vi "cfg combine v2 and v32.vi"(8 "error in":errorcluster, 10 "Log Actions":T1(array[cluster]), 11 "Engine Configuration In":T3(array[cluster])) -> (0 "error out":errorcluster, 3 "Engine Configuration Out":T4[](array[typedef]))   [LabVIEW 2013, in "Standard Engine Configuration.lvclass"]
uses:
  Standard Engine Configuration.lvclass
  Module Specific Configuration.ctl
  Module Decimation.ctl
  Runtime/error responses.ctl
  error options.ctl
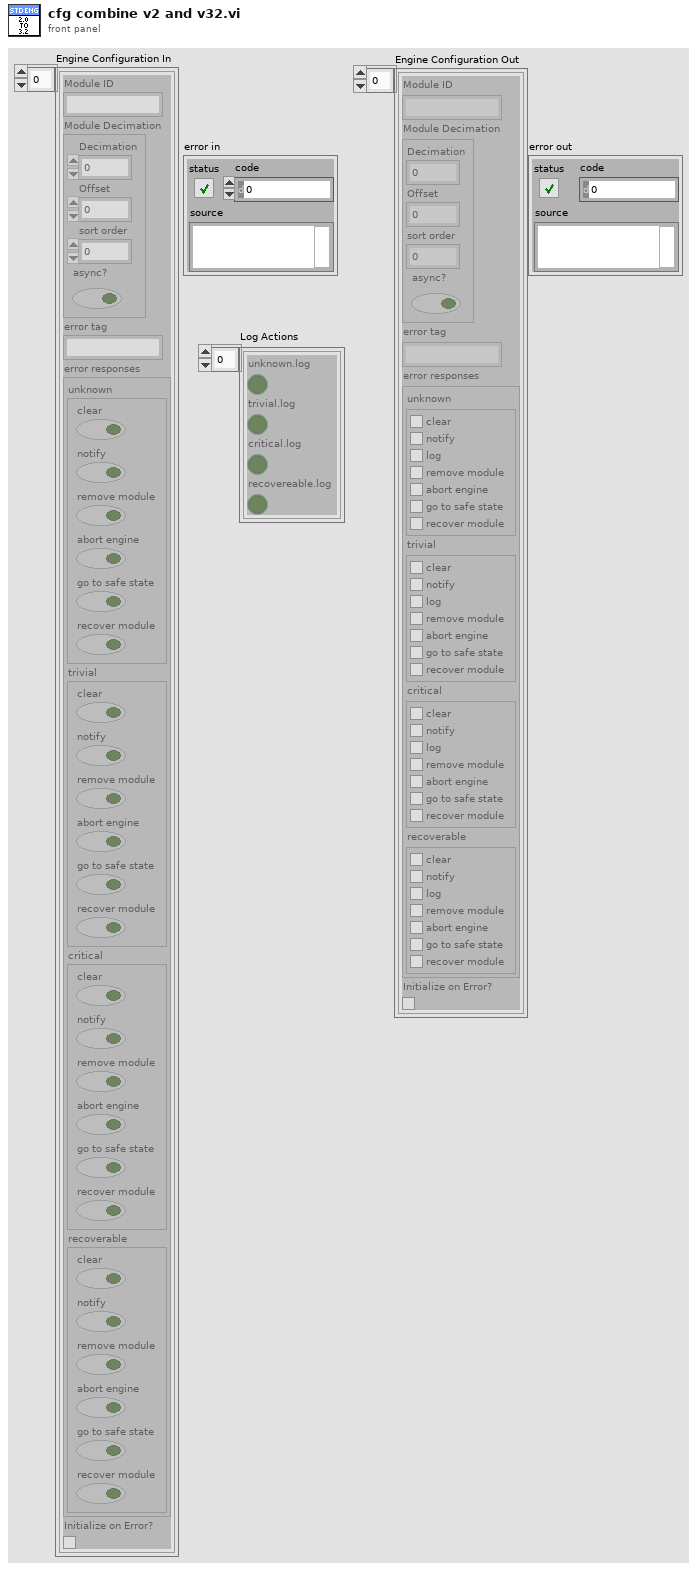
[diagram p1: front panel]
types:
  T1 = cluster{"unknown.log":bool, "trivial.log":bool, "critical.log":bool, "recovereable.log":bool}[]
  T2 = typedef "Standard Engine Configuration.lvclass/Module Decimation.ctl" = cluster{"Decimation":u16, "Offset":u16, "sort order":i32, "async?":bool}
  T3 = cluster{"Module ID":string, "Module Decimation":T2, "error tag":string, "error responses":cluster{"unknown":cluster{"clear":bool, "notify":bool, "remove module":bool, "abort engine":bool, "go to safe state":bool, "recover module":bool}, "trivial":cluster{"clear":bool, "notify":bool, "remove module":bool, "abort engine":bool, "go to safe state":bool, "recover module":bool}, "critical":cluster{"clear":bool, "notify":bool, "remove module":bool, "abort engine":bool, "go to safe state":bool, "recover module":bool}, "recoverable":cluster{"clear":bool, "notify":bool, "remove module":bool, "abort engine":bool, "go to safe state":bool, "recover module":bool}}, "Initialize on Error?":bool}[]
  T4 = typedef "Standard Engine Configuration.lvclass/Module Specific Configuration.ctl" = cluster{"Module ID":string, "Module Decimation":T2, "error tag":string, "error responses":T5, "Initialize on Error?":bool}
  T5 = typedef "Standard Engine Configuration.lvclass/error responses.ctl" = cluster{"unknown":T6, "trivial":T6, "critical":T6, "recoverable":T6}
  T6 = typedef "Standard Engine Configuration.lvclass/error options.ctl" = cluster{"clear":bool, "notify":bool, "log":bool, "remove module":bool, "abort engine":bool, "go to safe state":bool, "recover module":bool}
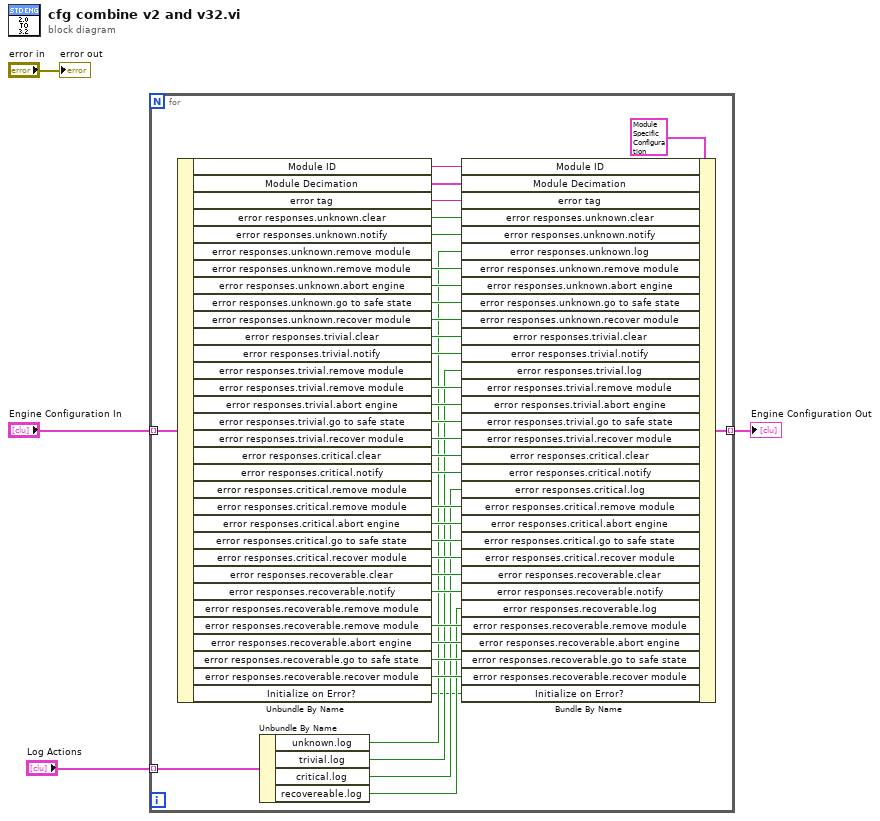
[diagram p0: block diagram]
diagram:
  n1 = for {
    tunnel: "Engine Configuration In" -> [w40] mode=indexing
    tunnel: [w38] -> w2 mode=indexing
    tunnel: "Log Actions" -> [w10] mode=indexing
    n2 = Unbundle By Name(w40) -> ("Module ID"=w37:string, "Module Decimation"=w36:T2, "error tag"=w35:string, "error responses.unknown.clear"=w34:bool, "error responses.unknown.notify"=w33:bool, "error responses.unknown.remove module"=w29:bool, "error responses.unknown.abort engine"=w30:bool, "error responses.unknown.go to safe state"=w32:bool, "error responses.unknown.recover module"=w31:bool, "error responses.trivial.clear"=w28:bool, "error responses.trivial.notify"=w27:bool, "error responses.trivial.remove module"=w26:bool, "error responses.trivial.abort engine"=w25:bool, "error responses.trivial.go to safe state"=w24:bool, "error responses.trivial.recover module"=w23:bool, "error responses.critical.clear"=w22:bool, "error responses.critical.notify"=w21:bool, "error responses.critical.remove module"=w20:bool, "error responses.critical.abort engine"=w19:bool, "error responses.critical.go to safe state"=w18:bool, "error responses.critical.recover module"=w17:bool, "error responses.recoverable.clear"=w16:bool, "error responses.recoverable.notify"=w15:bool, "error responses.recoverable.remove module"=w14:bool, "error responses.recoverable.abort engine"=w13:bool, "error responses.recoverable.go to safe state"=w12:bool, "error responses.recoverable.recover module"=w11:bool, "Initialize on Error?"=w5:bool)  [unwired: 4 out]
    n3 = Unbundle By Name(w10) -> ("unknown.log"=w9:bool, "trivial.log"=w8:bool, "critical.log"=w7:bool, "recovereable.log"=w6:bool)
    n4 = Bundle By Name(cluster=T4 {"Module ID"="", "Module Decimation"={"Decimation"=0, "Offset"=0, "sort order"=0, "async?"=FALSE}, "error tag"="", "error responses"={"unknown"={"clear"=FALSE, "notify"=FALSE, "log"=FALSE, "remove module"=FALSE, "abort engine"=FALSE, "go to safe state"=FALSE, "recover module"=FALSE}, "trivial"={"clear"=FALSE, "notify"=FALSE, "log"=FALSE, "remove module"=FALSE, "abort engine"=FALSE, "go to safe state"=FALSE, "recover module"=FALSE}, "critical"={"clear"=FALSE, "notify"=FALSE, "log"=FALSE, "remove module"=FALSE, "abort engine"=FALSE, "go to safe state"=FALSE, "recover module"=FALSE}, "recoverable"={"clear"=FALSE, "notify"=FALSE, "log"=FALSE, "remove module"=FALSE, "abort engine"=FALSE, "go to safe state"=FALSE, "recover module"=FALSE}}, "Initialize on Error?"=FALSE} ("Module Specific Configuration"), "Module ID"=w37, "Module Decimation"=w36, "error tag"=w35, "error responses.unknown.clear"=w34, "error responses.unknown.notify"=w33, "error responses.unknown.log"=w9, "error responses.unknown.remove module"=w29, "error responses.unknown.abort engine"=w30, "error responses.unknown.go to safe state"=w32, "error responses.unknown.recover module"=w31, "error responses.trivial.clear"=w28, "error responses.trivial.notify"=w27, "error responses.trivial.log"=w8, "error responses.trivial.remove module"=w26, "error responses.trivial.abort engine"=w25, "error responses.trivial.go to safe state"=w24, "error responses.trivial.recover module"=w23, "error responses.critical.clear"=w22, "error responses.critical.notify"=w21, "error responses.critical.log"=w7, "error responses.critical.remove module"=w20, "error responses.critical.abort engine"=w19, "error responses.critical.go to safe state"=w18, "error responses.critical.recover module"=w17, "error responses.recoverable.clear"=w16, "error responses.recoverable.notify"=w15, "error responses.recoverable.log"=w6, "error responses.recoverable.remove module"=w14, "error responses.recoverable.abort engine"=w13, "error responses.recoverable.go to safe state"=w12, "error responses.recoverable.recover module"=w11, "Initialize on Error?"=w5) -> (w38:T4)
  }
  "Engine Configuration Out" <- w2
  "error out" <- "error in"
